vi "timestampManifest.get.vi"(8 "error in (no error)":errorcluster, 11 "video in":refnum<class "video.lvclass">) -> (0 "error out":errorcluster, 2 "nominal types.lvlib:timestampManifest.lvlib:timestampManifest.lvclass":refnum<class "timestampManifest.lvclass">, 3 "video out":refnum<class "video.lvclass">)   [LabVIEW 2020, in "datasources.lvlib" / "video.lvclass"]
uses:
  video.lvclass
  nominal types/timestampManifest/timestampManifest/timestampManifest.lvclass
  video.lvclass/video.ctl
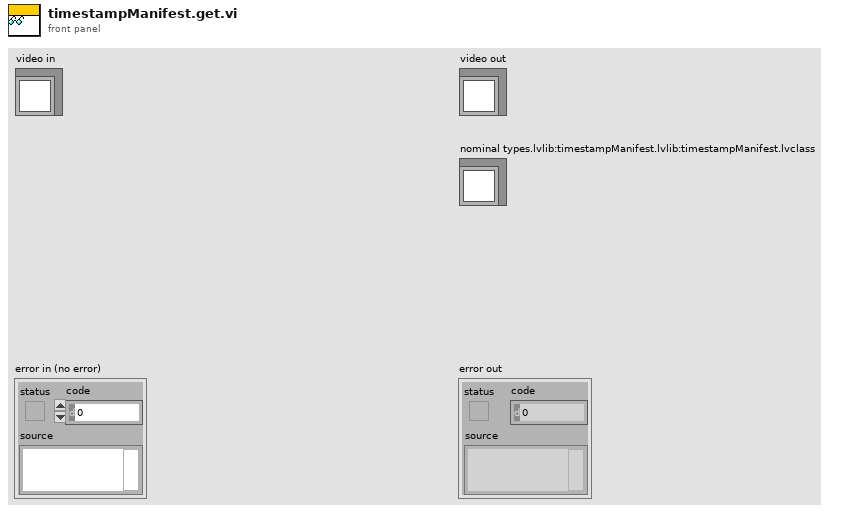
[diagram p1: front panel]
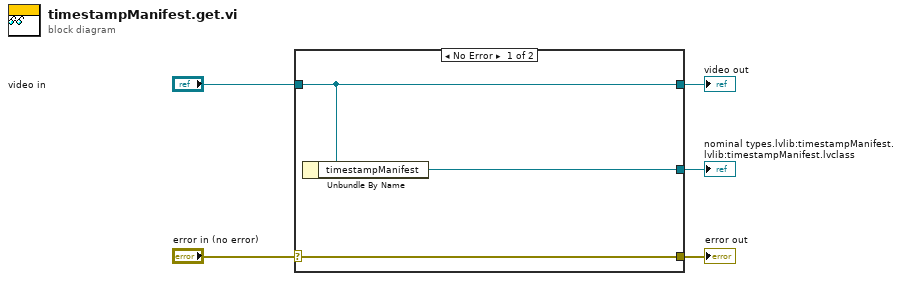
[diagram p0: block diagram]
diagram:
  n1 = case shown="No Error" "error in (no error)" {
    selector: "error in (no error)" -> [w8 w9]
    tunnel: [w8 w9] -> w4
    tunnel: [w7 w10] -> w2
    tunnel: "video in" -> [w7 w10]
    tunnel: [w6 _] -> w1
    frame No Error {
      n2 = Unbundle By Name(w7) -> ("timestampManifest"=w6:refnum<class "timestampManifest.lvclass">)
    }
    frame Error {
    }
  }
  "error out" <- w4
  "video out" <- w2
  "nominal types.lvlib:timestampManifest.lvlib:timestampManifest.lvclass" <- w1
